vi "Receive Control Mouse Down Event.vi"(8 "error in (no error)":errorcluster, 10 "ControlMouseDownMsg":refnum<class "ControlMouseDownMsg.lvclass">, 11 "TreeActor In":refnum<class "TreeActor.lvclass">) -> (0 "error out":errorcluster, 3 "TreeActor Out":refnum<class "TreeActor.lvclass">)   [LabVIEW 2015, in "TestViewables.lvlib" / "TreeActor.lvclass"]
doc: "<License>\nCopyright © 2017 Composed Systems, LLC | All rights reserved\nwww.composed.io\n\nAuthor: Ethan Stern <ethan.stern@composed.io>\n\nThis software is provided \"AS IS\" WITHOUT WARRANTIES, either express or implied, AND IS FOR EDUCATIONAL PURPOSES ONLY.\n</License>"
uses:
  TreeActor.lvclass
  Framework/ActorEvents/IEventAggregator Messages/ControlMouseDownMsg/ControlMouseDownMsg.lvclass
  Framework/ActorEvents/IEventAggregator Messages/ControlMouseDownMsg/ControlMouseDownMsg.lvclass/ControlMouseDownMsg.ctl
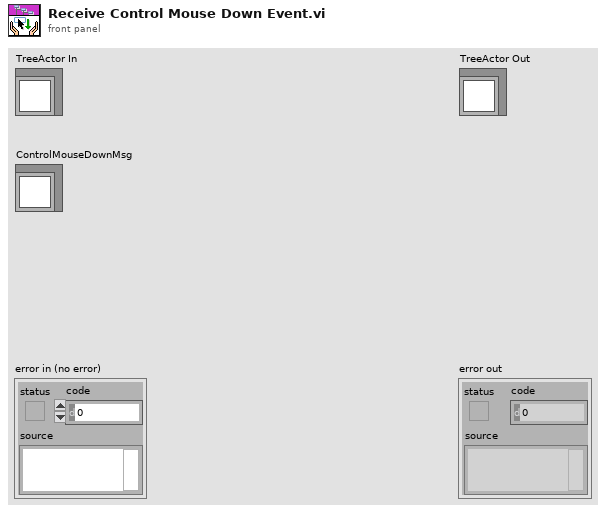
[diagram p1: front panel]
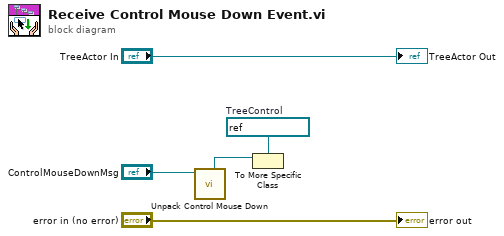
[diagram p0: block diagram]
diagram:
  w1 = refnum<vi> refnum  # TreeControl
  n1 = call "Unpack Control Mouse Down.vi"("ControlMouseDownMsg"="ControlMouseDownMsg") -> ("Ctl Refnum"=w2:refnum<vi>)  [unwired: 4 in, 6 out]
  n2 = To More Specific Class(target class=w1, reference=w2) -> ()  [unwired: 1 in, 2 out]
  "error out" <- "error in (no error)"
  "TreeActor Out" <- "TreeActor In"
